vi "Recall or Store Configuration.vi"(7 "Configuration ID (1: Block 1)":i32(ring)=1 items=["Block 1"=1, "Block 2"=2, "Block 3"=3, "Block 4"=4, "Block 5"=5, "Block 6"=6, "Block 7"=7, "Block 8"=8, "Block 9"=9, "Block 10"=10], 8 "error in (no error)":errorcluster, 9 "Store Configuration Name (\"Untitled1\")":string="Untitled1", 10 "Operation (0: Internal Recall)":i32(ring) items=["Internal Recall", "Internal Store"], 11 "VISA resource name":refnum<visa-resource-name>) -> (0 "error out":errorcluster, 3 "VISA resource name out":refnum<visa-resource-name>)   [LabVIEW 2020, in "Library Instrument & Equipement.lvlib" / "Library Power_Supply.lvlib" / "RIGOL DP800 Series.lvlib"]
doc: "Recalls or stores the instrument settings."
uses:
  RIGOL DP800 Series.lvlib
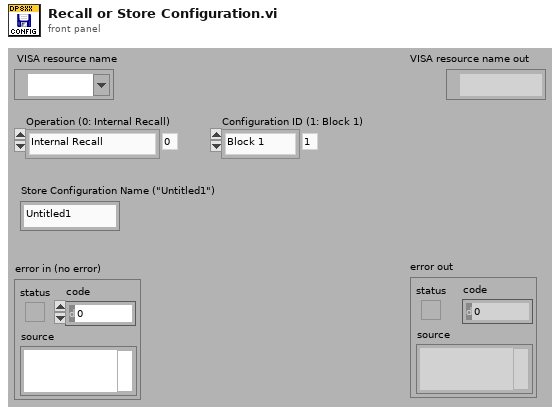
[diagram p1: front panel]
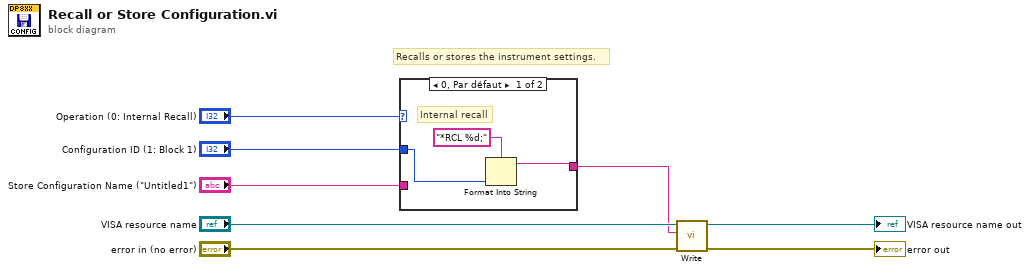
[diagram p0: block diagram]
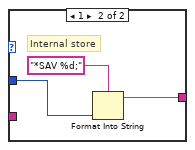
[diagram p2: hidden frame]
diagram:
  # "Recalls or stores the instrument settings."
  n1 = case shown="0, Par défaut" "Operation (0: Internal Recall)" {
    tunnel: "Configuration ID (1: Block 1)" -> [w11 w13]
    tunnel: "Store Configuration Name (\"Untitled1\")" -> [_ _]
    tunnel: [w9 w12] -> w1
    frame 0, Default {
      # "Internal recall"
      n2 = Format Into String(format string="*RCL %d;", w11) -> (resulting string=w9:string)  [unwired: 2 in, 1 out]
    }
    frame 1 {
      # "Internal store"
      n3 = Format Into String(format string="*SAV %d;", w13) -> (resulting string=w12:string)  [unwired: 2 in, 1 out]
    }
  }
  n4 = call "Write.vi"("error in (no error)"="error in (no error)", "Write Buffer (\"\")"=w1, "VISA resource name"="VISA resource name") -> ("error out"=→"error out":errorcluster, "VISA resource name out"=→"VISA resource name out":refnum<visa-resource-name>)  [unwired: 7 in]
